vi "Initialize.vi"(7 "LabPack Shared Library":path=path "", 8 "Error In":errorcluster) -> (0 "Error Out":errorcluster, 4 "Version":string)   [LabVIEW 2017, in "LabPack.lvlib"]
uses:
  LabPack.lvlib
  Private/Globals.vi
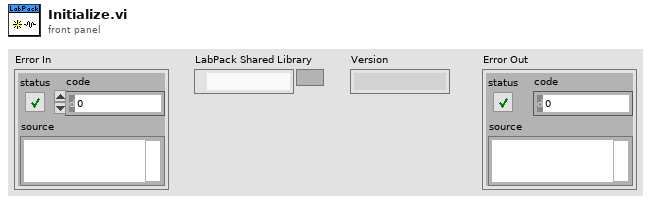
[diagram p1: front panel]
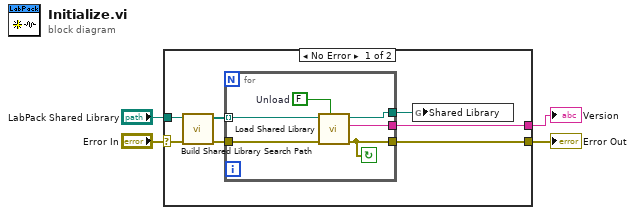
[diagram p0: block diagram]
diagram:
  n1 = case shown="No Error" "Error In" {
    selector: "Error In" -> [w9 w18]
    tunnel: "LabPack Shared Library" -> [w11 _]
    tunnel: [w10 w18] -> w3
    tunnel: [w8 _] -> w1
    frame No Error {
      n2 = call "Build Shared Library Search Path.vi"("Error In"=w9, "LabPack Shared Library"=w11) -> ("Error Out"=w7:errorcluster, "Search Path"=w6:path[])  [unwired: 8 in]
      n3 = for {
        tunnel: w7 -> [w17]
        tunnel: w6 -> [w14] mode=indexing
        tunnel: [w16] -> w10
        tunnel: [w15] -> w5
        tunnel: [w12] -> w8
        stop <- w16 continue-if-true
        w13 = FALSE  # Unload
        n4 = call "Load Shared Library.vi"("Unload"=w13, "Error In"=w17, "LabPack Shared Library In"=w14) -> ("Error Out"=w16:errorcluster, "Version"=w12:string, "LabPack Shared Library Out"=w15:path)  [unwired: 6 in]
      }
      n5 = global write "Globals.vi" "Shared Library"(w5) -> ()
    }
    frame Error {
    }
  }
  "Error Out" <- w3
  "Version" <- w1
